vi "2_Speech_Rec(Train).vi"() -> ()   [LabVIEW 2020]
doc: "This example demonstrates the usage of Deep Learning Toolkit for solving hand written digit recognition problem with Convolutional Neural Network (CNN).\n\nDataset: MNIST http://yann.lecun.com/exdb/mnist/\nRequirements: Deep Learning Toolkit for LabVIEW."
uses:
  <vilib>/Ngene/Deep Learning Toolkit/Toolkit/NN_Train/Controls/NN_Train_Params.ctl
  <vilib>/Ngene/Deep Learning Toolkit/Toolkit/NN_Train/Controls/NN_Train_Optimizer.ctl
  <vilib>/Ngene/Deep Learning Toolkit/Toolkit/NN_Train/Controls/NN_Train_Data_Sampling.ctl
  <vilib>/Ngene/Deep Learning Toolkit/Toolkit/NN_Train/Controls/NN_Train_Session_Data.ctl
  <vilib>/Ngene/Deep Learning Toolkit/Toolkit/NN_Train/Controls/NN_LR_Policy_Cfg.ctl
  <vilib>/Ngene/Deep Learning Toolkit/Toolkit/NN_Train/Controls/NN_LR_Policy_Type.ctl
  <vilib>/Ngene/Deep Learning Toolkit/Toolkit/NN_Network/Controls/NN_Device.ctl
  <vilib>/Ngene/Deep Learning Toolkit/Toolkit/NN_Network/Controls/NN_Save_Before_Destroy_Options.ctl
  <vilib>/Ngene/Deep Learning Toolkit/Toolkit/NN_Layers/Layers/Input/Controls/NN_Layer_Config(Input3D).ctl
  <vilib>/Ngene/Deep Learning Toolkit/Toolkit/NN_Data/API/NN_Dims(C,H,W).ctl
  <vilib>/Ngene/Deep Learning Toolkit/Toolkit/NN_Data/Controls/NN_Data_type.ctl
  <vilib>/Ngene/Deep Learning Toolkit/Toolkit/NN_Layers/Layers/FC/Controls/NN_Layer_Config(FC).ctl
  <vilib>/Ngene/Deep Learning Toolkit/Toolkit/NN_Layers/Layers/BatchNorm/Controls/NN_BN_Params.ctl
  <vilib>/Ngene/Deep Learning Toolkit/Toolkit/NN_Activations/Controls/NN_Activation_Type.ctl
  <vilib>/Ngene/Deep Learning Toolkit/Toolkit/NN_Layers/Controls/NN_Layer_Init_Params.ctl
  <vilib>/Ngene/Deep Learning Toolkit/Toolkit/NN_Layers/Controls/NN_Layer_Weight_Init_Type.ctl
  <vilib>/Ngene/Deep Learning Toolkit/Toolkit/NN_Layers/Layers/DropOut3D/Controls/NN_Layer_Config(DropOut3D).ctl
  <vilib>/Ngene/Deep Learning Toolkit/Toolkit/NN_Layers/Layers/Conv2D/Controls/NN_Layer_Config(Conv2D).ctl
  <vilib>/Ngene/Deep Learning Toolkit/Toolkit/NN_Layers/Layers/Conv2D/Controls/NN_Layer_Params(Conv2D).ctl
  <vilib>/Ngene/Deep Learning Toolkit/Toolkit/NN_Layers/Layers/Conv2D/Controls/NN_Conv2D_Padding_Type.ctl
  <vilib>/Ngene/Deep Learning Toolkit/Toolkit/NN_Layers/Layers/Input/NN_Layer_Create(Input3D).vi
  <vilib>/Ngene/Deep Learning Toolkit/Toolkit/NN_Layers/Layers/Conv2D/NN_Layer_Create(Conv2D).vi
  <vilib>/Ngene/Deep Learning Toolkit/Toolkit/NN_Layers/Layers/FC/NN_Layer_Create(FC).vi
  <vilib>/Ngene/Deep Learning Toolkit/Toolkit/NN_Layers/Layers/Dropout/NN_Layer_Create(DropOut).vi
  <vilib>/Ngene/Deep Learning Toolkit/Toolkit/NN_Layers/Layers/SoftMax/NN_Layer_Create(SoftMax).vi
  <vilib>/Ngene/Deep Learning Toolkit/Toolkit/NN_Train/Loss_Functions/NN_Set_Loss(CrossEntropy).vi
  <vilib>/Ngene/Deep Learning Toolkit/Toolkit/NN_Network/subVIs/NN_Predict/NN_Predict(In3D_Out1D).vi
  <vilib>/Ngene/Deep Learning Toolkit/Toolkit/NN_Train/Eval_Loss/NN_Eval_Test_Error_Loss/NN_Eval(In3D_Out1D).vi
  <vilib>/Ngene/Deep Learning Toolkit/Toolkit/NN_Train/Eval_Loss/NN_Calc_Cofusion_Matrix/NN_Calc_Confusion_Matrix(In3D_Out1D).vi
  <vilib>/Ngene/Deep Learning Toolkit/Toolkit/NN_Data/subVIs/Dataset_Destroy/NN_Datasets_All_Destroy(In3D_Out1D).vi
  <vilib>/Ngene/Deep Learning Toolkit/Toolkit/Deep_Learning_Toolkit_by_Ngene.lvlib
  <vilib>/ptbypt/NI_PtbyPt.lvlib
panel:
  in  "Tab":enum32{"Training", "Confusion Matrix"}(tab)
  out "Train/Test Metrics":T1={"Train_Loss"=0.286125585064292, "Test_Loss"=0.3077670633792877, "Test_Error"=0.09372638165950775} {"Test_Error" format="%#_4g"; "Test_Loss" format="%#_4g"; "Train_Loss" format="%#_4g"}
  in  "Dataset Path(Test)":path=path ""
  out "Train Speed (s/iter)":dbl=6084.864852491099 format="%#_3p"
  out "Train Graphs":T2(graph)={"mean"=0.286125585064292, "Valid_Loss"=0.30776706, "Valid_Error"=0.09372638}
  in  "Eval Test":bool
  out "Session Data":T3={"Epochs"=9.183652, "Tot_Iter"=6834, "LR"=0.0625, "LR_iter"=6835}
  in  "Stop":bool
  in  "LR Update Policy":T4={"Policy_Type"=enum."Step", "LR0"=0.5, "k"=3.0, "WarmUp_Policy"=enum."Ramp", "WarmUp_Iter"=500, "WarmUp_Ratio"=10.0} {"WarmUp_Ratio" min=1; "WarmUp_Iter" min=1; "LR0" format="%.7f"}
  out "Train Speed (s/iter)":dbl=0.0210357999894768 format="%#_2p"
  in  "Train_Params":T6={"Optimizer"=enum."SGD", "Beta_1"=0.9, "Beta_2"=0.999, "Weight Decay(L1)"=5e-07, "Weight Decay(L2)"=5e-07, "Data_Sampling"=enum."Random"}
  out "Time_Elapsed":dbl=186.16946299999836 format="%<%H:%M:%S>t"
  in  "Working Dir":path=path "D:/working"
  in  "Dataset Path(Train)":path=path "D:/Data/DNN/Speech_Commands/data_speech_commands_v0.02_stft"
  in  "NN_Device":T9=enum."GPU"
  out "Generated Trained Model Files":path[](array[path])=[path "D:/working/Speech_Rec/Speech_Rec_net_cfg_26_07_10__17_58_19.cfg", path "D:/working/Speech_Rec/Speech_Rec_weights_26_07_10__17_58_19.bin", path "D:/working/Speech_Rec/Speech_Rec_render_26_07_10__17_58_19.svg"]
  out "Confusion Matrix":string[][](table)=[["0", "0", "0", "0", "0", "0", "0", "0", "0", "0", "0", "0", "0", "0", "0", "0", "0", "0", "0", "0", "0", "0", "0", "0", "0", "0", "0", "0", "0", "0", "0", "0", "0", "0", "0", "0", "NaN"], ["0", "145", "5", "1", "0", "0", "0", "0", "1", "0", "2", "0", "1", "1", "0", "0", "1", "1", "0", "1", "1", "0", "1", "0", "2", "0", "0", "0", "0", "0", "1", "0", "2", "0", "0", "0", "0.8735"], ["0", "0", "181", "3", "3", "0", "0", "3", "0", "0", "0", "0", "0", "1", "0", "0", "9", "0", "4", "1", "0", "0", "0", "3", "0", "0", "0", "0", "0", "0", "0", "1", "2", "0", "1", "0", "0.8538"], ["0", "0", "6", "191", "0", "2", "1", "0", "1", "0", "0", "0", "0", "0", "0", "0", "0", "0", "0", "2", "0", "0", "0", "3", "0", "0", "0", "0", "0", "0", "1", "0", "1", "0", "1", "1", "0.9095"], ["0", "0", "2", "1", "176", "0", "4", "0", "0", "0", "0", "0", "0", "1", "1", "0", "0", "0", "0", "1", "0", "0", "0", "0", "0", "0", "1", "1", "0", "1", "3", "1", "0", "0", "2", "0", "0.9026"], ["0", "1", "2", "2", "0", "189", "9", "0", "0", "0", "0", "0", "5", "0", "0", "0", "0", "0", "3", "7", "0", "0", "0", "1", "0", "0", "0", "0", "0", "0", "2", "0", "0", "0", "0", "0", "0.8552"], ["0", "0", "1", "0", "4", "1", "363", "0", "0", "0", "0", "0", "3", "0", "0", "0", "0", "1", "2", "6", "0", "3", "0", "0", "3", "0", "0", "1", "0", "0", "4", "0", "0", "0", "0", "0", "0.9260"], ["0", "0", "1", "0", "1", "0", "0", "378", "1", "0", "0", "0", "0", "1", "4", "0", "1", "0", "0", "0", "0", "3", "0", "2", "0", "0", "1", "0", "1", "1", "2", "0", "1", "0", "0", "1", "0.9474"], ["0", "0", "0", "1", "1", "0", "0", "0", "364", "3", "0", "0", "2", "1", "3", "0", "1", "3", "2", "0", "1", "6", "2", "1", "1", "0", "0", "0", "0", "0", "1", "6", "0", "0", "0", "0", "0.9123"], ["0", "0", "0", "0", "0", "0", "0", "1", "3", "144", "13", "4", "5", "0", "1", "0", "0", "1", "0", "0", "1", "3", "0", "0", "1", "0", "0", "0", "0", "0", "0", "1", "0", "0", "0", "0", "0.8090"], ["0", "0", "0", "0", "0", "0", "0", "0", "1", "2", "135", "17", "1", "0", "1", "0", "0", "1", "1", "0", "0", "3", "0", "0", "1", "0", "0", "0", "0", "0", "0", "1", "0", "0", "0", "0", "0.8232"], ["0", "1", "0", "1", "1", "2", "0", "0", "2", "2", "11", "337", "7", "0", "2", "0", "1", "0", "0", "0", "2", "1", "0", "0", "1", "0", "0", "1", "0", "0", "2", "1", "0", "0", "0", "0", "0.8987"], ["0", "0", "0", "1", "2", "8", "11", "0", "0", "0", "2", "4", "299", "0", "0", "0", "0", "1", "0", "25", "0", "0", "0", "0", "0", "0", "0", "1", "1", "0", "5", "2", "1", "0", "0", "2", "0.8192"], ["0", "0", "0", "0", "1", "0", "1", "0", "0", "0", "0", "0", "0", "178", "2", "0", "0", "0", "0", "0", "0", "0", "0", "1", "0", "0", "0", "0", "0", "0", "1", "3", "0", "0", "0", "0", "0.9519"], ["0", "0", "0", "0", "0", "0", "0", "0", "0", "0", "0", "0", "0", "5", "198", "0", "0", "1", "0", "1", "3", "3", "0", "0", "0", "0", "0", "0", "0", "0", "0", "2", "0", "0", "0", "0", "0.9296"], ["0", "0", "0", "2", "0", "2", "4", "0", "0", "0", "0", "1", "1", "0", "0", "120", "2", "0", "5", "5", "0", "0", "1", "1", "0", "1", "0", "0", "0", "0", "1", "0", "1", "1", "3", "0", "0.7947"], ["0", "1", "1", "0", "1", "0", "0", "1", "0", "0", "0", "1", "0", "1", "0", "2", "348", "0", "2", "0", "1", "0", "1", "0", "0", "0", "0", "0", "0", "0", "1", "1", "2", "0", "6", "0", "0.9405"], ["0", "0", "0", "0", "0", "0", "0", "0", "1", "0", "0", "0", "0", "1", "1", "0", "1", "197", "7", "0", "0", "1", "2", "0", "0", "0", "1", "0", "0", "1", "0", "1", "1", "1", "0", "0", "0.9120"], ["0", "3", "2", "1", "0", "1", "1", "1", "3", "0", "0", "0", "0", "0", "0", "2", "1", "4", "325", "3", "0", "2", "2", "0", "0", "0", "0", "0", "0", "0", "0", "2", "0", "0", "0", "0", "0.9207"], ["0", "0", "2", "1", "0", "3", "12", "0", "0", "0", "0", "0", "13", "0", "0", "4", "0", "0", "6", "324", "0", "0", "0", "0", "1", "0", "0", "0", "2", "0", "1", "0", "0", "0", "1", "0", "0.8757"], ["0", "0", "1", "0", "1", "1", "0", "0", "1", "4", "0", "1", "1", "0", "3", "0", "0", "1", "0", "0", "348", "4", "0", "0", "0", "0", "1", "0", "0", "1", "2", "11", "0", "0", "0", "0", "0.9134"], ["0", "0", "1", "0", "0", "0", "1", "1", "1", "3", "0", "2", "3", "0", "1", "0", "0", "0", "0", "0", "4", "345", "5", "0", "0", "0", "1", "0", "0", "0", "0", "2", "0", "0", "0", "0", "0.9324"], ["0", "0", "0", "0", "0", "1", "1", "0", "0", "1", "0", "1", "1", "0", "0", "3", "3", "2", "1", "0", "0", "7", "366", "3", "0", "0", "0", "0", "1", "0", "0", "1", "0", "3", "0", "0", "0.9266"], ["0", "0", "2", "2", "0", "0", "2", "1", "6", "0", "0", "0", "1", "1", "0", "1", "8", "0", "4", "0", "0", "0", "2", "368", "0", "0", "1", "1", "0", "0", "0", "0", "0", "0", "0", "0", "0.9200"], ["0", "1", "0", "0", "0", "0", "1", "0", "1", "3", "0", "0", "1", "0", "0", "0", "0", "1", "0", "0", "2", "2", "0", "0", "393", "2", "4", "3", "1", "0", "2", "0", "0", "0", "0", "1", "0.9402"], ["0", "0", "0", "0", "1", "0", "0", "0", "0", "0", "0", "1", "0", "0", "0", "0", "0", "1", "0", "0", "0", "0", "0", "0", "1", "174", "0", "1", "1", "0", "1", "0", "0", "0", "1", "6", "0.9255"], ["0", "0", "0", "1", "0", "0", "0", "3", "0", "0", "0", "0", "1", "0", "0", "0", "1", "0", "0", "0", "0", "0", "0", "0", "1", "0", "344", "0", "0", "1", "3", "0", "0", "0", "1", "2", "0.9609"], ["0", "0", "0", "0", "1", "3", "2", "0", "0", "0", "0", "2", "2", "0", "1", "0", "0", "0", "0", "0", "2", "1", "0", "0", "1", "0", "0", "369", "0", "0", "2", "10", "0", "0", "0", "0", "0.9318"], ["0", "1", "0", "2", "1", "0", "0", "6", "0", "0", "0", "0", "1", "0", "0", "1", "0", "0", "0", "0", "2", "0", "0", "1", "1", "1", "0", "0", "323", "29", "8", "0", "1", "0", "0", "5", "0.8433"], ["0", "0", "0", "0", "0", "0", "0", "3", "0", "0", "0", "0", "0", "0", "1", "0", "0", "0", "0", "0", "1", "0", "0", "0", "1", "0", "1", "1", "30", "130", "6", "0", "0", "0", "0", "1", "0.7429"], ["0", "0", "0", "0", "0", "0", "0", "4", "0", "0", "0", "0", "1", "0", "0", "0", "0", "0", "0", "1", "0", "1", "0", "0", "1", "3", "1", "1", "6", "1", "375", "1", "0", "0", "0", "2", "0.9422"], ["0", "0", "0", "0", "0", "0", "1", "0", "1", "1", "0", "1", "2", "3", "3", "0", "0", "0", "0", "1", "13", "4", "0", "0", "0", "0", "0", "2", "1", "1", "2", "370", "0", "0", "0", "0", "0.9113"], ["0", "0", "0", "0", "0", "0", "0", "0", "0", "0", "0", "0", "0", "0", "0", "0", "0", "0", "0", "1", "0", "0", "0", "0", "0", "1", "1", "0", "2", "0", "1", "0", "158", "0", "1", "1", "0.9518"], ["0", "0", "0", "0", "1", "1", "2", "0", "1", "1", "0", "0", "2", "0", "0", "2", "1", "0", "1", "3", "1", "1", "13", "0", "0", "0", "0", "0", "0", "0", "0", "1", "0", "166", "0", "0", "0.8426"], ["0", "0", "0", "0", "2", "0", "0", "0", "1", "0", "0", "0", "0", "0", "0", "0", "9", "0", "1", "1", "0", "0", "0", "0", "0", "0", "2", "0", "0", "0", "2", "0", "0", "1", "376", "1", "0.9495"], ["0", "0", "0", "0", "0", "0", "0", "0", "0", "0", "0", "0", "2", "0", "0", "1", "0", "0", "0", "1", "0", "0", "0", "0", "2", "2", "0", "1", "0", "1", "11", "0", "2", "0", "1", "397", "0.9430"], ["NaN", "0.9477", "0.8744", "0.9095", "0.8934", "0.8832", "0.8726", "0.9403", "0.9357", "0.8780", "0.8282", "0.9059", "0.8423", "0.9175", "0.8919", "0.8824", "0.8992", "0.9163", "0.8929", "0.8437", "0.9110", "0.8846", "0.9266", "0.9583", "0.9562", "0.9457", "0.9582", "0.9634", "0.8753", "0.7784", "0.8523", "0.8852", "0.9186", "0.9651", "0.9543", "0.9452", ""]]
  out "Test_Error(Final)":sgl=0.09353741
  out "Test_Loss(Final)":sgl=0.30383846 format="%#_3g"
  out "Test_Error":sgl=0.09372638
  out "Test_Loss":sgl=0.30776706
  # "5. Observe the training speed.\n6. Periodically press the \"Eval Test\" button to evaluate the Validation Loss/Error. Note that validation error evaluation influences the training speed, as the forward network inference is run for the whole validation dataset.\n7. Hit the \"Stop Train\" button when the Test Loss/Error is no longer decreasing.\n8. Observe the Test_Error(Final) value - this represents the final accuracy of the trained network.\n9. The Paths of the ttrained model will be provided in \"Generated Trained Model Files\".\n10. Deployment: For deployment, please open \"3_Speech_Rec_Deploy(file).vi\" or \"4_Speech_Rec_Deploy(mic).vi\".\n\nMore Examples: https://github.com/ngenehub/deepltk_examples"
  # "Overview: This example demonstrates the use of Deep Learning Toolkit for solving a speech recognition problem.\nRequirements:\n- Deep Learning Toolkit for LabVIEW.\n- NI Vision Development Module.\nInstructions:\n1. Provide the path to the image dataset generated in the previous step at the \"Dataset Path (Train)\" control.\n2. Set the appropriate path at the \"Working Dir\" control, where the trained model will be stored.\n3. Run the VI with the current configuration of the training parameters and Learning Rate update policy.\n4. Observe how the training loss decreases."
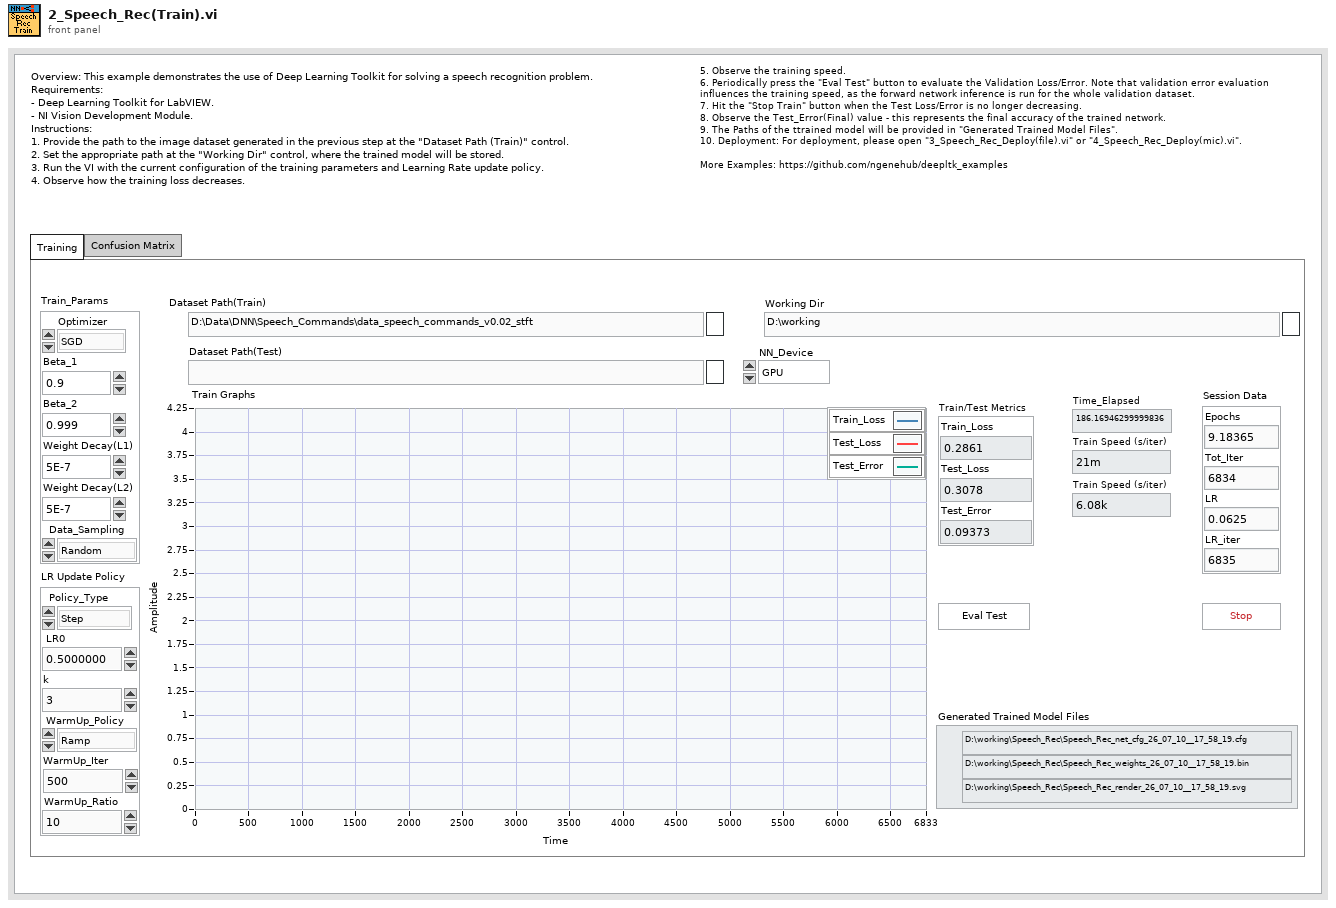
[diagram p1: front panel]
types:
  T1 = cluster{"Train_Loss":dbl, "Test_Loss":dbl, "Test_Error":dbl}
  T2 = cluster{"mean":dbl, "Valid_Loss":sgl, "Valid_Error":sgl}
  T3 = typedef "Deep_Learning_Toolkit_by_Ngene.lvlib/NN_Train_Session_Data.ctl" = cluster{"Epochs":sgl, "Tot_Iter":i32, "LR":sgl, "LR_iter":i32}
  T4 = typedef "Deep_Learning_Toolkit_by_Ngene.lvlib/NN_LR_Policy_Cfg.ctl" = cluster{"Policy_Type":T5, "LR0":dbl, "k":sgl, "WarmUp_Policy":enum16{"Step", "Ramp"}, "WarmUp_Iter":i32, "WarmUp_Ratio":sgl}
  T5 = typedef "Deep_Learning_Toolkit_by_Ngene.lvlib/NN_LR_Policy_Type.ctl" = enum16{"Manual", "Step", "Exp", "1/t"}
  T6 = typedef "Deep_Learning_Toolkit_by_Ngene.lvlib/NN_Train_Params.ctl" = cluster{"Optimizer":T7, "Beta_1":sgl, "Beta_2":sgl, "Weight Decay(L1)":sgl, "Weight Decay(L2)":sgl, "Data_Sampling":T8}
  T7 = typedef "Deep_Learning_Toolkit_by_Ngene.lvlib/NN_Train_Optimizer.ctl" = enum16{"SGD", "Adam", "Adagrad", "Adadelta", "RMSProp", "Nesterov"}
  T8 = typedef "Deep_Learning_Toolkit_by_Ngene.lvlib/NN_Train_Data_Sampling.ctl" = enum16{"Random", "Sequential"}
  T9 = typedef "Deep_Learning_Toolkit_by_Ngene.lvlib/NN_Device.ctl" = enum16{"CPU", "GPU"}
  T10 = typedef "Deep_Learning_Toolkit_by_Ngene.lvlib/NN_Layer_Config(Conv2D).ctl" = cluster{"Name":string, "Conv_Params":T11, "BN?":bool, "BN_Params":T13, "Activation":T14, "Has Bias?":bool, "Init_Params":T15, "Custom_Params":string}
  T11 = typedef "Deep_Learning_Toolkit_by_Ngene.lvlib/NN_Layer_Params(Conv2D).ctl" = cluster{"Filters":i32, "Kernel_Size":i32, "Stride":i32, "Pad_Type":T12, "Pad_Size":i32}
  T12 = typedef "Deep_Learning_Toolkit_by_Ngene.lvlib/NN_Conv2D_Padding_Type.ctl" = enum16{"Pad_Size", "Valid", "Same"}
  T13 = typedef "Deep_Learning_Toolkit_by_Ngene.lvlib/NN_BN_Params.ctl" = cluster{"epsilon":sgl, "momentum":sgl}
  T14 = typedef "Deep_Learning_Toolkit_by_Ngene.lvlib/NN_Activation_Type.ctl" = enum16{"Sigmoid", "ReLU", "LReLU", "ReLU6", "GELU", "tanh", "Swish", "Mish", "None"}
  T15 = typedef "Deep_Learning_Toolkit_by_Ngene.lvlib/NN_Layer_Init_Params.ctl" = cluster{"Init_Type":T16, "Value":sgl}
  T16 = typedef "Deep_Learning_Toolkit_by_Ngene.lvlib/NN_Layer_Weight_Init_Type.ctl" = enum16{"Const", "Uniform", "Gaussian", "Xavier"}
  T17 = typedef "Deep_Learning_Toolkit_by_Ngene.lvlib/NN_Layer_Config(DropOut3D).ctl" = cluster{"Name":string, "Probability":sgl}
  T18 = typedef "Deep_Learning_Toolkit_by_Ngene.lvlib/NN_Layer_Config(FC).ctl" = cluster{"Name":string, "Size":i32, "BN":bool, "BN_Params":T13, "Activation":T14, "Has Bias?":bool, "Init_Params":T15, "Custom_Params":string}
  T19 = typedef "Deep_Learning_Toolkit_by_Ngene.lvlib/NN_Layer_Config(Input3D).ctl" = cluster{"Name":string, "Dims":T20, "Data_Type":T21, "Shifts":sgl[], "Scales":sgl[]}
  T20 = typedef "Deep_Learning_Toolkit_by_Ngene.lvlib/NN_Dims(C,H,W).ctl" = cluster{"C":i32, "H":i32, "W":i32}
  T21 = typedef "Deep_Learning_Toolkit_by_Ngene.lvlib/NN_Data_type.ctl" = enum16{"I8", "U8", "I16", "U16", "U32 ARGB", "SGL"}
  T22 = typedef "Deep_Learning_Toolkit_by_Ngene.lvlib/NN_Save_Before_Destroy_Options.ctl" = cluster{"CFG?":bool, "Weights?":bool, "Render?":bool}
  T23 = typedef "Deep_Learning_Toolkit_by_Ngene.lvlib/NN_DataSets_All(In3D_Out1D).ctl" = cluster{"Train":T24, "Validation":T24, "Test":T24}
  T24 = typedef "Deep_Learning_Toolkit_by_Ngene.lvlib/NN_DataSet(In3D_Out1D).ctl" = cluster{"Inputs Ref.":variant, "Outputs Ref.":T25, "Dataset_Size":i32, "Dims_In":T20, "Dims_Out":i32, "Labels":string[], "File Paths":path[], "Custom_Data":variant}
  T25 = typedef "Deep_Learning_Toolkit_by_Ngene.lvlib/NN_Data_ref(2D_SGL).ctl" = refnum<data-value>
  T26 = typedef "Deep_Learning_Toolkit_by_Ngene.lvlib/NN.ctl" = cluster{"Name":string, "No of Layers":i32, "mBatch":i32, "Layers":T27[], "Dimty":T28, "Dims_In":T20, "Dims_Out":T20, "Working_Dir":path, "Train?":bool, "Train_Params":T6, "LR_Update_Policy":T4, "Session Data":T3, "Ground_truth":T29, "NNg_hdls":T30, "NN_Device":T9, "GPU Id":i32, "Labels":string[], "Loss_Type":T31, "Loss_Cfg_Prms":variant, "NNG_WS":T32, "DryRun?":bool}
  T27 = typedef "Deep_Learning_Toolkit_by_Ngene.lvlib/NN_Layer_ref.ctl" = refnum<file>
  T28 = typedef "Deep_Learning_Toolkit_by_Ngene.lvlib/NN_In_Out_Dim-ty.ctl" = enum8{"In1D_Out1D", "In3D_Out1D", "In3D_Out3D", "In3D_OutBBox"}
  T29 = typedef "Deep_Learning_Toolkit_by_Ngene.lvlib/NN_Ground_truth.ctl" = cluster{"Y":variant}
  T30 = typedef "Deep_Learning_Toolkit_by_Ngene.lvlib/nng_cuda_handles.ctl" = cluster{"cudnn":u64, "cublas":u64, "stream":u64, "curand":u64}
  T31 = typedef "Deep_Learning_Toolkit_by_Ngene.lvlib/NN_Loss_Type.ctl" = enum16{"None", "MSE", "CrossEntropy", "YOLO_v2", "YOLO_v4"}
  T32 = typedef "Deep_Learning_Toolkit_by_Ngene.lvlib/NNG_WS.ctl" = cluster{"NNG_WS_Mem":T33, "Max_WS_Size":i64}
  T33 = typedef "Deep_Learning_Toolkit_by_Ngene.lvlib/NNg_WS_Mem_DVR.ctl" = refnum<data-value>
  T34 = typedef "Deep_Learning_Toolkit_by_Ngene.lvlib/NN_Eval_Params.ctl" = cluster{"Loss":sgl, "Error":sgl}
  T35 = cluster{"mean":dbl, "Test_Loss":sgl, "Test_Error":sgl}
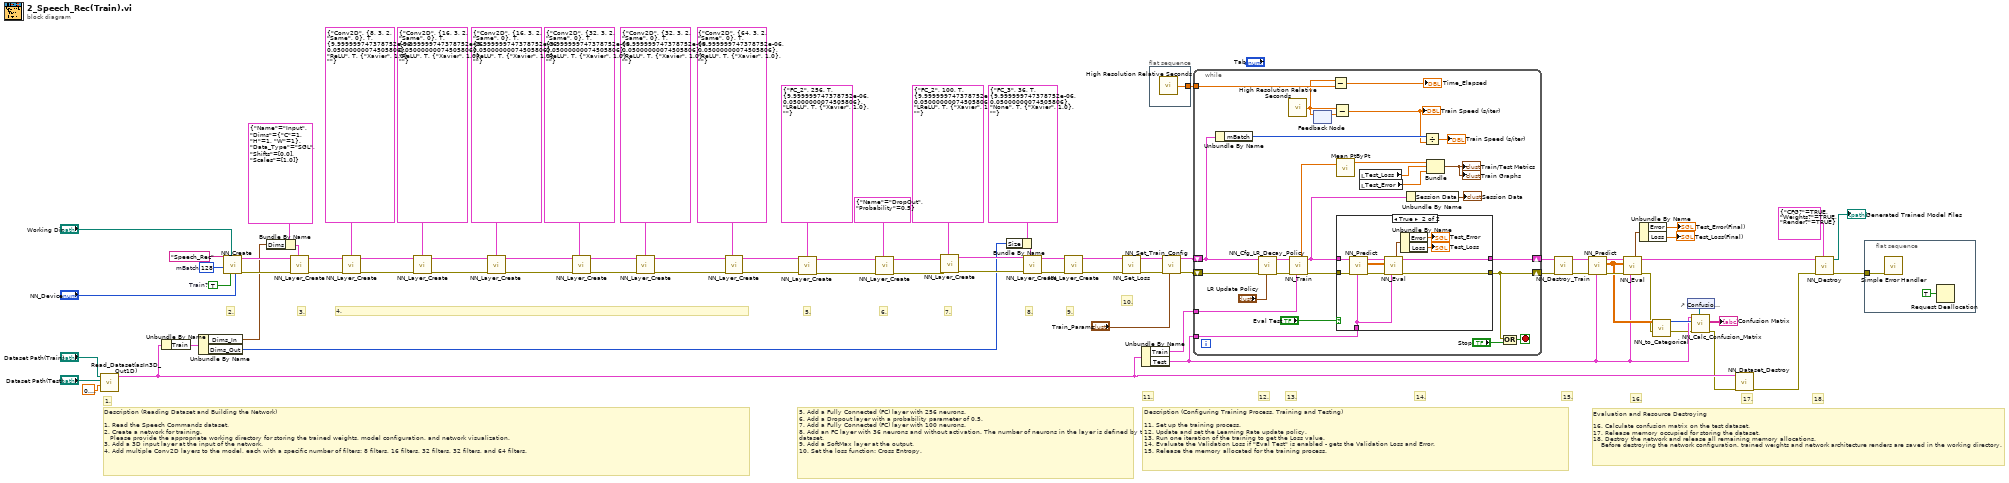
[diagram p0: block diagram]
diagram:
  w48 = TRUE  # Train?
  w53 = 128  # mBatch
  # "14."
  # "13."
  # "12."
  # "Description (Configuring Training Process, Training and Testing)\n\n11. Set up the training process.\n12. Update and set the Learning Rate update policy.\n13. Run one iteration of the training to get the Loss value.\n14. Evaluate the Validation Loss if \"Eval Test\" is enabled - gets the Validation Loss and Error.\n15. Release the memory allocated for the training process."
  # "11."
  # "5. Add a Fully Connected (FC) layer with 256 neurons.\n6. Add a Dropout layer with a probability parameter of 0.5.\n7. Add a Fully Connected (FC) layer with 100 neurons.\n8. Add an FC layer with 36 neurons and without activation. The number of neurons in the layer is defined by the dataset.\n9. Add a SoftMax layer at the output.\n10. Set the loss function: Cross Entropy."
  # "Description (Reading Dataset and Building the Network)\n\n1. Read the Speech Commands dataset.\n2. Create a network for training.\n   Please provide the appropriate working directory for storing the trained weights, model configuration, and network visualization.\n3. Add a 3D input layer at the input of the network.\n4. Add multiple Conv2D layers to the model, each with a specific number of filters: 8 filters, 16 filters, 32 filters, 32 filters, and 64 filters."
  # "1."
  # "10."
  # "9."
  # "8."
  # "7."
  # "6."
  # "5."
  # "4."
  # "3."
  # "2."
  # "Evaluation and Resource Destroying\n\n16. Calculate confusion matrix on the test dataset.\n17. Release memory occupied for storing the dataset.\n18. Destroy the network and release all remaining memory allocations.\n    Before destroying the network configuration, trained weights and network architecture renders are saved in the working directory."
  # "18."
  # "15."
  # "17."
  # "16."
  n1 = call "Read_Dataset(asIn3D_Out1D).vi"("Validtn Split"=sgl 0.1 ("Valid_data_Size"), "Dataset Path(Test)"="Dataset Path(Test)", "Dataset Path(Train)"="Dataset Path(Train)") -> ("Datasets"=w75:T23)  [unwired: 7 in, 1 out]
  n2 = Unbundle By Name(w75) -> ("Train"=w74:T24)
  n3 = Unbundle By Name(w74) -> ("Dims_In"=w19:T20, "Dims_Out"=w18:i32)
  n4 = call <vilib>:"NN_Create.vi"("NN_Device"="NN_Device", "Train? (false)"=w48, "Working Dir"="Working Dir", "mBatch (1)"=w53, "Name"="Speech_Rec") -> ("error out"=w54:errorcluster, "NN out"=w55:T26)  [unwired: 5 in]
  n5 = Bundle By Name(cluster=T19 {"Name"="Input", "Dims"={"C"=1, "H"=1, "W"=1}, "Data_Type"=enum."SGL", "Shifts"=[0.0], "Scales"=[1.0]} ("Cluster"), "Dims"=w19) -> (w49:T19)
  n6 = call-poly <vilib>:"NN_Layer_Create.vi"("Input3D_Cfg"=w49, "error in (no error)"=w54, "NN In"=w55) -> ("error out"=w51:errorcluster, "NN out"=w52:T26)  [unwired: 6 in, 1 out]
  n7 = call-poly <vilib>:"NN_Layer_Create.vi"("Conv2D_Cfg"=T10 {"Name"="Conv2D", "Conv_Params"={"Filters"=8, "Kernel_Size"=3, "Stride"=2, "Pad_Type"=enum."Same", "Pad_Size"=0}, "BN?"=TRUE, "BN_Params"={"epsilon"=1e-05, "momentum"=0.05}, "Activation"=enum."ReLU", "Has Bias?"=TRUE, "Init_Params"={"Init_Type"=enum."Xavier", "Value"=1.0}, "Custom_Params"=""}, "error in (no error)"=w51, "NN in"=w52) -> ("error out"=w39:errorcluster, "NN out"=w40:T26)  [unwired: 6 in, 1 out]
  n8 = call-poly <vilib>:"NN_Layer_Create.vi"("Conv2D_Cfg"=T10 {"Name"="Conv2D", "Conv_Params"={"Filters"=16, "Kernel_Size"=3, "Stride"=2, "Pad_Type"=enum."Same", "Pad_Size"=0}, "BN?"=TRUE, "BN_Params"={"epsilon"=1e-05, "momentum"=0.05}, "Activation"=enum."ReLU", "Has Bias?"=TRUE, "Init_Params"={"Init_Type"=enum."Xavier", "Value"=1.0}, "Custom_Params"=""}, "error in (no error)"=w39, "NN in"=w40) -> ("error out"=w37:errorcluster, "NN out"=w38:T26)  [unwired: 6 in, 1 out]
  n9 = call-poly <vilib>:"NN_Layer_Create.vi"("Conv2D_Cfg"=T10 {"Name"="Conv2D", "Conv_Params"={"Filters"=16, "Kernel_Size"=3, "Stride"=2, "Pad_Type"=enum."Same", "Pad_Size"=0}, "BN?"=TRUE, "BN_Params"={"epsilon"=1e-05, "momentum"=0.05}, "Activation"=enum."ReLU", "Has Bias?"=TRUE, "Init_Params"={"Init_Type"=enum."Xavier", "Value"=1.0}, "Custom_Params"=""}, "error in (no error)"=w37, "NN in"=w38) -> ("error out"=w35:errorcluster, "NN out"=w36:T26)  [unwired: 6 in, 1 out]
  n10 = call-poly <vilib>:"NN_Layer_Create.vi"("Conv2D_Cfg"=T10 {"Name"="Conv2D", "Conv_Params"={"Filters"=32, "Kernel_Size"=3, "Stride"=2, "Pad_Type"=enum."Same", "Pad_Size"=0}, "BN?"=TRUE, "BN_Params"={"epsilon"=1e-05, "momentum"=0.05}, "Activation"=enum."ReLU", "Has Bias?"=TRUE, "Init_Params"={"Init_Type"=enum."Xavier", "Value"=1.0}, "Custom_Params"=""}, "error in (no error)"=w35, "NN in"=w36) -> ("error out"=w33:errorcluster, "NN out"=w34:T26)  [unwired: 6 in, 1 out]
  n11 = call-poly <vilib>:"NN_Layer_Create.vi"("Conv2D_Cfg"=T10 {"Name"="Conv2D", "Conv_Params"={"Filters"=32, "Kernel_Size"=3, "Stride"=2, "Pad_Type"=enum."Same", "Pad_Size"=0}, "BN?"=TRUE, "BN_Params"={"epsilon"=1e-05, "momentum"=0.05}, "Activation"=enum."ReLU", "Has Bias?"=TRUE, "Init_Params"={"Init_Type"=enum."Xavier", "Value"=1.0}, "Custom_Params"=""}, "error in (no error)"=w33, "NN in"=w34) -> ("error out"=w41:errorcluster, "NN out"=w42:T26)  [unwired: 6 in, 1 out]
  n12 = call-poly <vilib>:"NN_Layer_Create.vi"("Conv2D_Cfg"=T10 {"Name"="Conv2D", "Conv_Params"={"Filters"=64, "Kernel_Size"=3, "Stride"=2, "Pad_Type"=enum."Same", "Pad_Size"=0}, "BN?"=TRUE, "BN_Params"={"epsilon"=1e-05, "momentum"=0.05}, "Activation"=enum."ReLU", "Has Bias?"=TRUE, "Init_Params"={"Init_Type"=enum."Xavier", "Value"=1.0}, "Custom_Params"=""}, "error in (no error)"=w41, "NN in"=w42) -> ("error out"=w44:errorcluster, "NN out"=w45:T26)  [unwired: 6 in, 1 out]
  n13 = call-poly <vilib>:"NN_Layer_Create.vi"("FC_Cfg"=T18 {"Name"="FC_2", "Size"=256, "BN"=TRUE, "BN_Params"={"epsilon"=1e-05, "momentum"=0.05}, "Activation"=enum."LReLU", "Has Bias?"=TRUE, "Init_Params"={"Init_Type"=enum."Xavier", "Value"=1.0}, "Custom_Params"=""} ("Layer_Config_Params"), "error in (no error)"=w44, "NN in"=w45) -> ("error out"=w28:errorcluster, "NN out"=w30:T26)  [unwired: 6 in, 1 out]
  n14 = call-poly <vilib>:"NN_Layer_Create.vi"("DropOut_Cfg"=T17 {"Name"="DropOut", "Probability"=0.5}, "error in (no error)"=w28, "NN in"=w30) -> ("error out"=w27:errorcluster, "NN out"=w29:T26)  [unwired: 6 in, 1 out]
  n15 = call-poly <vilib>:"NN_Layer_Create.vi"("FC_Cfg"=T18 {"Name"="FC_2", "Size"=100, "BN"=TRUE, "BN_Params"={"epsilon"=1e-05, "momentum"=0.05}, "Activation"=enum."LReLU", "Has Bias?"=TRUE, "Init_Params"={"Init_Type"=enum."Xavier", "Value"=1.0}, "Custom_Params"=""} ("Layer_Config_Params"), "error in (no error)"=w27, "NN in"=w29) -> ("error out"=w46:errorcluster, "NN out"=w47:T26)  [unwired: 6 in, 1 out]
  n16 = Bundle By Name(cluster=T18 {"Name"="FC_3", "Size"=36, "BN"=TRUE, "BN_Params"={"epsilon"=1e-05, "momentum"=0.05}, "Activation"=enum."None", "Has Bias?"=TRUE, "Init_Params"={"Init_Type"=enum."Xavier", "Value"=1.0}, "Custom_Params"=""} ("Layer_Config_Params"), "Size"=w18) -> (w8:T18)
  n17 = call-poly <vilib>:"NN_Layer_Create.vi"("FC_Cfg"=w8, "error in (no error)"=w46, "NN in"=w47) -> ("error out"=w31:errorcluster, "NN out"=w32:T26)  [unwired: 6 in, 1 out]
  n18 = call-poly <vilib>:"NN_Layer_Create.vi"("error in (no error)"=w31, "NN in"=w32) -> ("error out"=w25:errorcluster, "NN out"=w26:T26)  [unwired: 7 in, 1 out]
  n19 = call-poly <vilib>:"NN_Set_Loss.vi"("error in (no error)"=w25, "NN in"=w26) -> ("error out"=w24:errorcluster, "NN out"=w23:T26)  [unwired: 8 in]
  n20 = Unbundle By Name(w75) -> ("Train"=w5:T24, "Test"=w56:T24)
  n21 = flat-sequence {
    tunnel: [w80] -> w78
    frame #0 {
      n22 = call <vilib>:"High Resolution Relative Seconds.vi"() -> ("relative seconds"=w80:dbl)
    }
  }
  n23 = call <vilib>:"NN_Set_Train_Config.vi"("NN_Train_Params"="Train_Params", "error in (no error)"=w24, "NN in"=w23) -> ("error out"=w21:errorcluster, "NN out"=w22:T26)  [unwired: 7 in]
  n24 = while {
    shift-right: [w89] -> w70
    shift-left: w21 -> [w83]
    shift-right: [w86] -> w71
    shift-left: w22 -> [w84]
    tunnel: w78 -> [w98]
    tunnel: w5 -> [w88]
    tunnel: w56 -> [w82]
    stop <- w105 stop-if-true
    n25 = Unbundle By Name(w84) -> ("mBatch"=w94:i32)
    n26 = call <vilib>:"NN_Cfg_LR_Decay_Policy.vi"("LR_Decay_Params"="LR Update Policy", "error in (no error)"=w83, "NN in"=w84) -> ("error out"=w100:errorcluster, "NN out"=w106:T26)  [unwired: 7 in]
    n27 = call <vilib>:"High Resolution Relative Seconds.vi"() -> ("relative seconds"=w97:dbl)
    n28 = call <vilib>:"NN_Train.vi"("Train Dataset"=w88, "error in (no error)"=w100, "NN in"=w106) -> ("error out"=w90:errorcluster, "NN out"=w85:T26, "Loss"=w101:sgl)  [unwired: 3 in, 3 out]
    n29 = feedback #1() -> (w107:dbl)  [unwired: 1 in]
    n30 = feedback-in #1(w97) -> ()
    n31 = Subtract(x=w97, y=w98) -> (x-y=→"Time_Elapsed":dbl)
    n32 = Subtract(x=w97, y=w107) -> (x-y=w92:dbl)
    "Train Speed (s/iter)" <- w92
    n33 = call <vilib>:"Mean PtByPt.vi"("x"=w101) -> ("mean"=w102:dbl)  [unwired: 3 in, 1 out]
    n34 = case shown="True" "Eval Test" {
      tunnel: w85 -> [w108 w120]
      tunnel: w90 -> [w109 w116]
      tunnel: [w109 w118] -> w89
      tunnel: [w108 w119] -> w86
      tunnel: w82 -> [_ w113]
      frame False {
      }
      frame True {
        n35 = call-poly <vilib>:"NN_Predict.vi"("Dataset"=w113, "error in (no error)"=w116, "NN in"=w120) -> ("error out"=w115:errorcluster, "Predictions"=w114:sgl[][], "NN out"=w117:T26)  [unwired: 6 in]
        n36 = call-poly <vilib>:"NN_Eval.vi"("Dataset"=w113, "error in (no error)"=w115, "Predictions"=w114, "NN in"=w117) -> ("error out"=w118:errorcluster, "NN out"=w119:T26, "NN_Eval_Params"=w112:T34)  [unwired: 4 in, 1 out]
        n37 = Unbundle By Name(w112) -> ("Error"=→"Test_Error":sgl, "Loss"=→"Test_Loss":sgl)
      }
    }
    n38 = local read "Test_Loss"() -> (w104:sgl)
    n39 = local read "Test_Error"() -> (w99:sgl)
    n40 = Unbundle By Name(w85) -> ("Session Data"=→"Session Data":T3)
    n41 = Divide(x=w94, y=w92) -> (x/y=→"Train Speed (s/iter)":dbl)
    n42 = Bundle("mean"=w102, "Test_Loss"=w104, "Test_Error"=w99) -> (→"Train Graphs" →"Train/Test Metrics":T35)  [unwired: 1 in]
    n43 = Compound Arithmetic op=OR(w89, "Stop") -> (w105:bool)
  }
  n44 = call <vilib>:"NN_Destroy_Train.vi"("error in (no error)"=w70, "NN in"=w71) -> ("error out"=w67:errorcluster, "NN out"=w69:T26)  [unwired: 8 in]
  n45 = call-poly <vilib>:"NN_Predict.vi"("Dataset"=w56, "error in (no error)"=w67, "NN in"=w69) -> ("error out"=w66:errorcluster, "Predictions"=w64:sgl[][], "NN out"=w68:T26)  [unwired: 6 in]
  n46 = call-poly <vilib>:"NN_Eval.vi"("Dataset"=w56, "error in (no error)"=w66, "Predictions"=w64, "NN in"=w68) -> ("error out"=w17:errorcluster, "NN out"=w57:T26, "NN_Eval_Params"=w60:T34)  [unwired: 4 in, 1 out]
  n47 = Unbundle By Name(w60) -> ("Error"=→"Test_Error(Final)":sgl, "Loss"=→"Test_Loss(Final)":sgl)
  n48 = call <vilib>:"NN_to_Categorical.vi"("Prediction"=w64) -> ("Label_Idx"=w65:i32[])  [unwired: 10 in]
  n49 = control-ref of="Confusion Matrix"() -> (w72:refnum<vi>)
  n50 = call-poly <vilib>:"NN_Calc_Confusion_Matrix.vi"("Confusion Matrix (Table) ref."=w72, "error in (no error)"=w17, "Predictions"=w65, "Dataset"=w56) -> ("error out"=w63:errorcluster, "Confusion Matrix (Table)"=→"Confusion Matrix":string[][])  [unwired: 3 in, 3 out]
  n51 = call-poly <vilib>:"NN_Dataset_Destroy.vi"("error in (no error)"=w63, "Datasets_All(In3D_Out1D)"=w75) -> ("error out"=w77:errorcluster)  [unwired: 9 in]
  n52 = call <vilib>:"NN_Destroy.vi"("Save (T, T, T)"=T22 {"CFG?"=TRUE, "Weights?"=TRUE, "Render?"=TRUE} ("Save_Config"), "error in (no error)"=w77, "NN in"=w57) -> ("error out"=w79:errorcluster, "Generated_Files"=→"Generated Trained Model Files":path[])  [unwired: 7 in]
  n53 = flat-sequence {
    tunnel: w79 -> [w122]
    frame #0 {
      n54 = call <vilib>:"Simple Error Handler.vi"("error in (no error)"=w122) -> ()  [unwired: 4 in, 5 out]
      n55 = Request Deallocation(TRUE ("flag")) -> ()
    }
  }
